vi "例题7.1.vi"() -> ()   [LabVIEW 2017]
panel:
  out "波形图 7":cluster{i32, i32, cluster{dbl[]}[]}(graph)
  out "波形图 6":cluster{i32, i32, dbl[][]}(graph)
  out "波形图 5":cluster{i32, i32, dbl[]}[](graph)
  out "波形图 4":cluster{i32, i32, dbl[]}(graph)
  out "波形图 3":cluster{dbl[]}[](graph)
  out "波形图 2":dbl[][](graph)
  out "波形图":dbl[](graph)
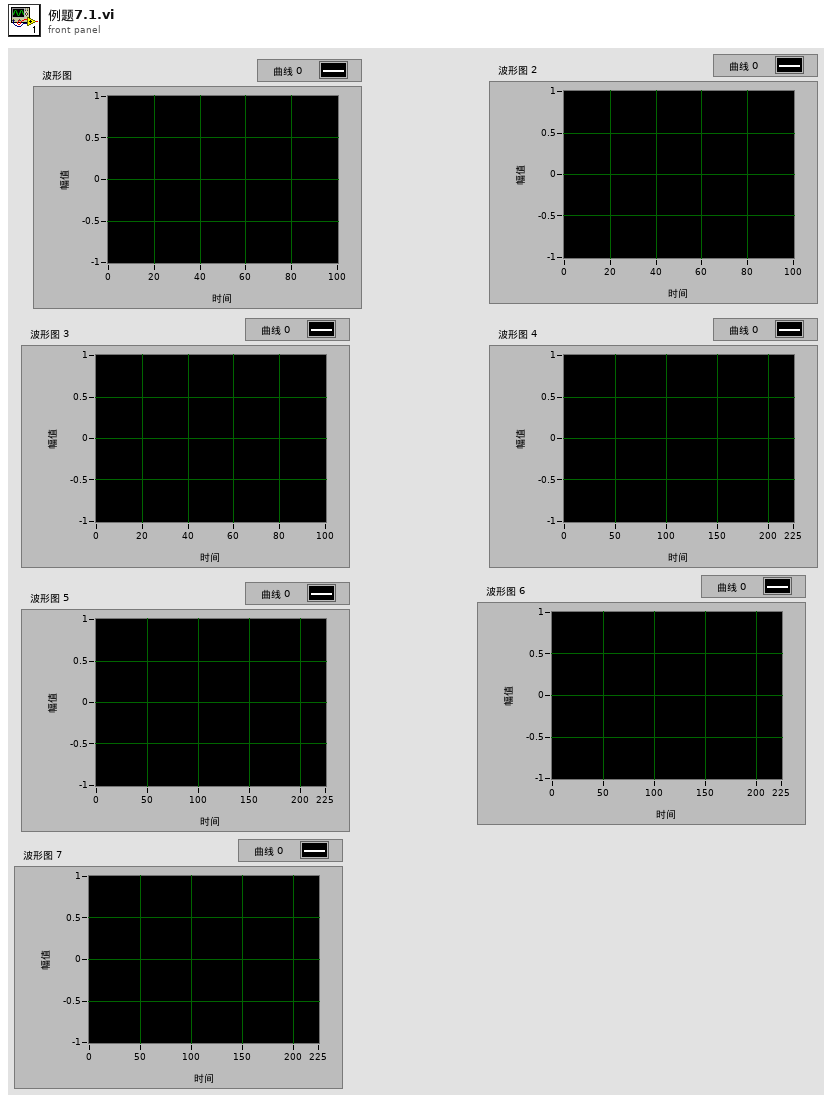
[diagram p1: front panel]
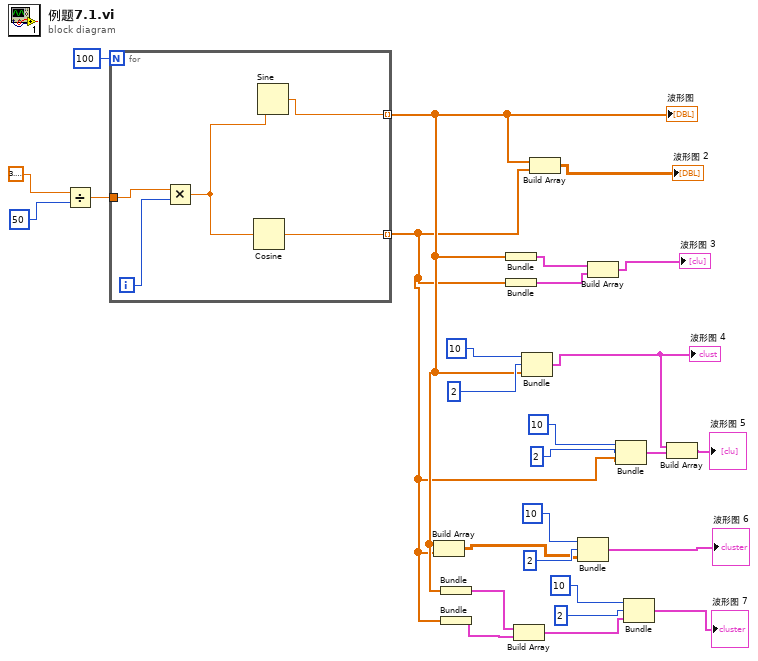
[diagram p0: block diagram]
diagram:
  n1 = Divide(x=3.141592653589793, y=50) -> (x/y=w24:dbl)
  n2 = for {
    N: 100 -> [_]
    tunnel: w24 -> [w31]
    tunnel: [w29] -> w8 mode=indexing
    tunnel: [w28] -> w7 mode=indexing
    i -> [w32]
    n3 = Multiply(x=w31, y=w32) -> (x*y=w30:dbl)
    n4 = Cosine(x=w30) -> (cos(x)=w28:dbl)
    n5 = Sine(x=w30) -> (sin(x)=w29:dbl)
  }
  "波形图" <- w8
  n6 = Build Array(w8, w7) -> (w10:dbl[][])
  n7 = Bundle(w8) -> (w6:cluster{dbl[]})  [unwired: 1 in]
  n8 = Bundle(w7) -> (w5:cluster{dbl[]})  [unwired: 1 in]
  n9 = Bundle(w8) -> (w23:cluster{dbl[]})  [unwired: 1 in]
  n10 = Bundle(w7) -> (w22:cluster{dbl[]})  [unwired: 1 in]
  n11 = Build Array(w6, w5) -> (w2:cluster{dbl[]}[])
  n12 = Bundle(10, 2, w8) -> (w13:cluster{i32, i32, dbl[]})  [unwired: 1 in]
  "波形图 4" <- w13
  n13 = Build Array(w8, w7) -> (→"波形图 2":dbl[][])
  n14 = Bundle(10, 2, w10) -> (→"波形图 6":cluster{i32, i32, dbl[][]})  [unwired: 1 in]
  n15 = Build Array(w23, w22) -> (→"波形图 3":cluster{dbl[]}[])
  n16 = Bundle(10, 2, w7) -> (w14:cluster{i32, i32, dbl[]})  [unwired: 1 in]
  n17 = Bundle(10, 2, w2) -> (→"波形图 7":cluster{i32, i32, cluster{dbl[]}[]})  [unwired: 1 in]
  n18 = Build Array(w13, w14) -> (→"波形图 5":cluster{i32, i32, dbl[]}[])
